vi "HW Stop.vi"(8 "error in (no error)":errorcluster) -> (0 "error out":errorcluster)   [LabVIEW 2017]
uses:
  Global Variables/General Globals.vi
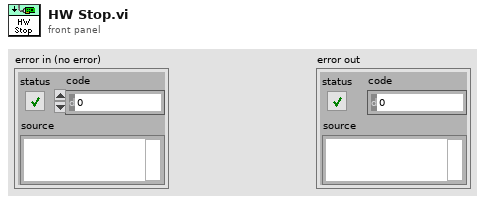
[diagram p1: front panel]
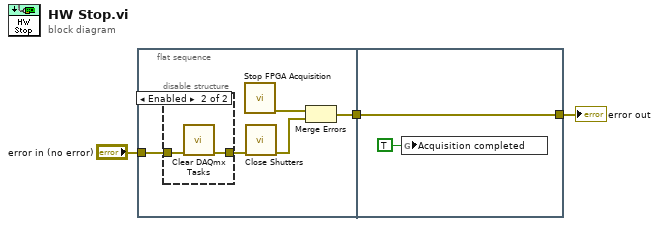
[diagram p0: block diagram]
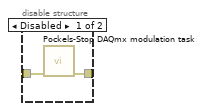
[diagram p2: hidden frame]
diagram:
  n1 = flat-sequence {
    tunnel: "error in (no error)" -> [w4]
    tunnel: [w8] -> w1
    tunnel: [w14] -> w3
    tunnel: w1 -> [w14]
    frame #0 {
      n2 = disable-structure shown="Enabled" {
        disable-tunnel: [w10 w11] -> w5
        disable-tunnel: w4 -> [w9 w12]
        frame Disabled {
          n3 = call "Pockels-Stop DAQmx modulation task.vi"("error in"=w9) -> ("error out"=w10:errorcluster)  [unwired: 10 in]
        }
        frame Enabled {
          n4 = call "Clear DAQmx Tasks.vi"("error in (no error)"=w12) -> ("error out"=w11:errorcluster)  [unwired: 10 in]
        }
      }
      n5 = call "Stop FPGA Acquisition.vi"() -> ("Error Out"=w7:errorcluster)  [unwired: 10 in, 1 out]
      n6 = call "Close Shutters.vi"("error in (no error)"=w5) -> ("error out (no error)"=w6:errorcluster)  [unwired: 10 in]
      n7 = Merge Errors(w7, w6) -> (w8:errorcluster)
    }
    frame #1 {
      n8 = global write "General Globals.vi" "Acquisition completed"(TRUE ("Acquisition completed")) -> ()
    }
  }
  "error out" <- w3
